vi "Read UserEvent Ref.vi"(8 "error in":errorcluster, 11 "UserEventMessageTransport in":refnum<class "UserEventMessageTransport.lvclass">) -> (0 "error out":errorcluster, 2 "UserEvent Ref":refnum<user-event>, 3 "UserEventMessageTransport out":refnum<class "UserEventMessageTransport.lvclass">)   [LabVIEW 2016, in "UserEventMessageTransport.lvclass"]
uses:
  UserEventMessageTransport.lvclass
  IMessagePayload/IMessagePayload.lvclass
  UserEventMessageTransport.lvclass/UserEventMessageTransport.ctl
panel:
  # "INPUTS"
  # "OUTPUTS"
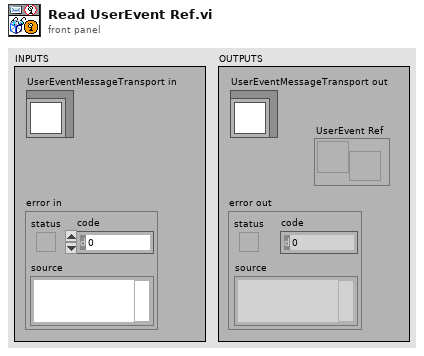
[diagram p1: front panel]
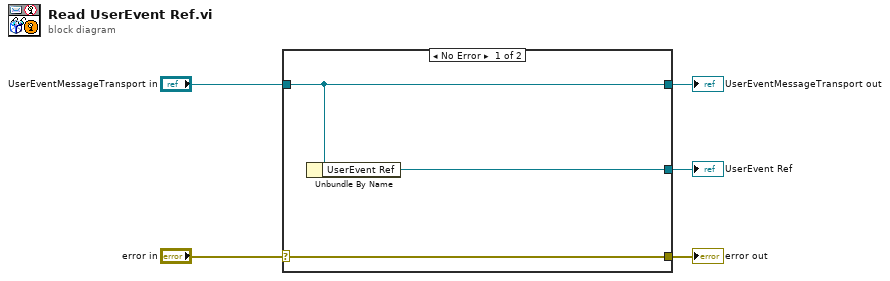
[diagram p0: block diagram]
diagram:
  n1 = case shown="No Error" "error in" {
    selector: "error in" -> [w8 w9]
    tunnel: [w8 w9] -> w4
    tunnel: [w7 w10] -> w2
    tunnel: "UserEventMessageTransport in" -> [w7 w10]
    tunnel: [w6 _] -> w1
    frame No Error {
      n2 = Unbundle By Name(w7) -> ("UserEvent Ref"=w6:refnum<user-event>)
    }
    frame Error {
    }
  }
  "error out" <- w4
  "UserEventMessageTransport out" <- w2
  "UserEvent Ref" <- w1
